vi "code-generator.vi"() -> ()   [LabVIEW 2014]
uses:
  <vilib>/addons/Digital Filter Design/_Objects.llb/DFD Quantization Settings.ctl
  <vilib>/addons/Digital Filter Design/_Objects.llb/DFD Quantization Sources.ctl
  <vilib>/addons/Digital Filter Design/FXPModel.llb/DFD FXP Quantize Coef (Easy).vi
  <vilib>/addons/Digital Filter Design/Process.llb/DFD Filtering (Wfm).vi
  <vilib>/addons/Digital Filter Design/FXPLib.llb/DFD FXP to I16 (scalar).vi
  <vilib>/addons/Digital Filter Design/CodeGen.llb/DFD FXP C Code Generator.vi
  <vilib>/Utility/VariantDataType/GetNumericFxpInfo.vi
  <vilib>/addons/Digital Filter Design/FXPSim.llb/dfd_Check Input FXP Settings.vi
  <vilib>/addons/Digital Filter Design/FXPSim.llb/dfd_Check SRate Simulation Integer Input.vi
  <vilib>/addons/Digital Filter Design/FXPSim.llb/dfd_FXP Simu.vi
  <vilib>/addons/Digital Filter Design/_Objects.llb/DFD FXP Statistics Data.ctl
  <vilib>/addons/Digital Filter Design/FXPSim.llb/SimXnode/DFD FXP Simulation.xnode
  <vilib>/addons/Digital Filter Design/_Objects.llb/DFD Filter Obj.ctl
  <vilib>/addons/Digital Filter Design/_Objects.llb/DFD Filter Coef.ctl
  <vilib>/addons/Digital Filter Design/_Objects.llb/DFD Filter Structure Type Selector.ctl
  <vilib>/addons/Digital Filter Design/_Objects.llb/dfd_Internal Quantization Settings.ctl
  <vilib>/addons/Digital Filter Design/_Objects.llb/dfd_Internal Quantization Srcs.ctl
  <vilib>/addons/Digital Filter Design/_Objects.llb/DFD Coef Norm Type.ctl
  <vilib>/addons/Digital Filter Design/NI_DigFilterLicensed.lvlib
  <vilib>/measure/NI_MABase.lvlib
  <vilib>/addons/Digital Filter Design/NI_DigFilter_FXP.lvlib
  <vilib>/Utility/VariantDataType/VariantType.lvlib
panel:
  out "output files":path[](array[path])
  out "coefficients report":string
  out "filtering text report":string
  out "signal out":waveform(dbl)[](graph)
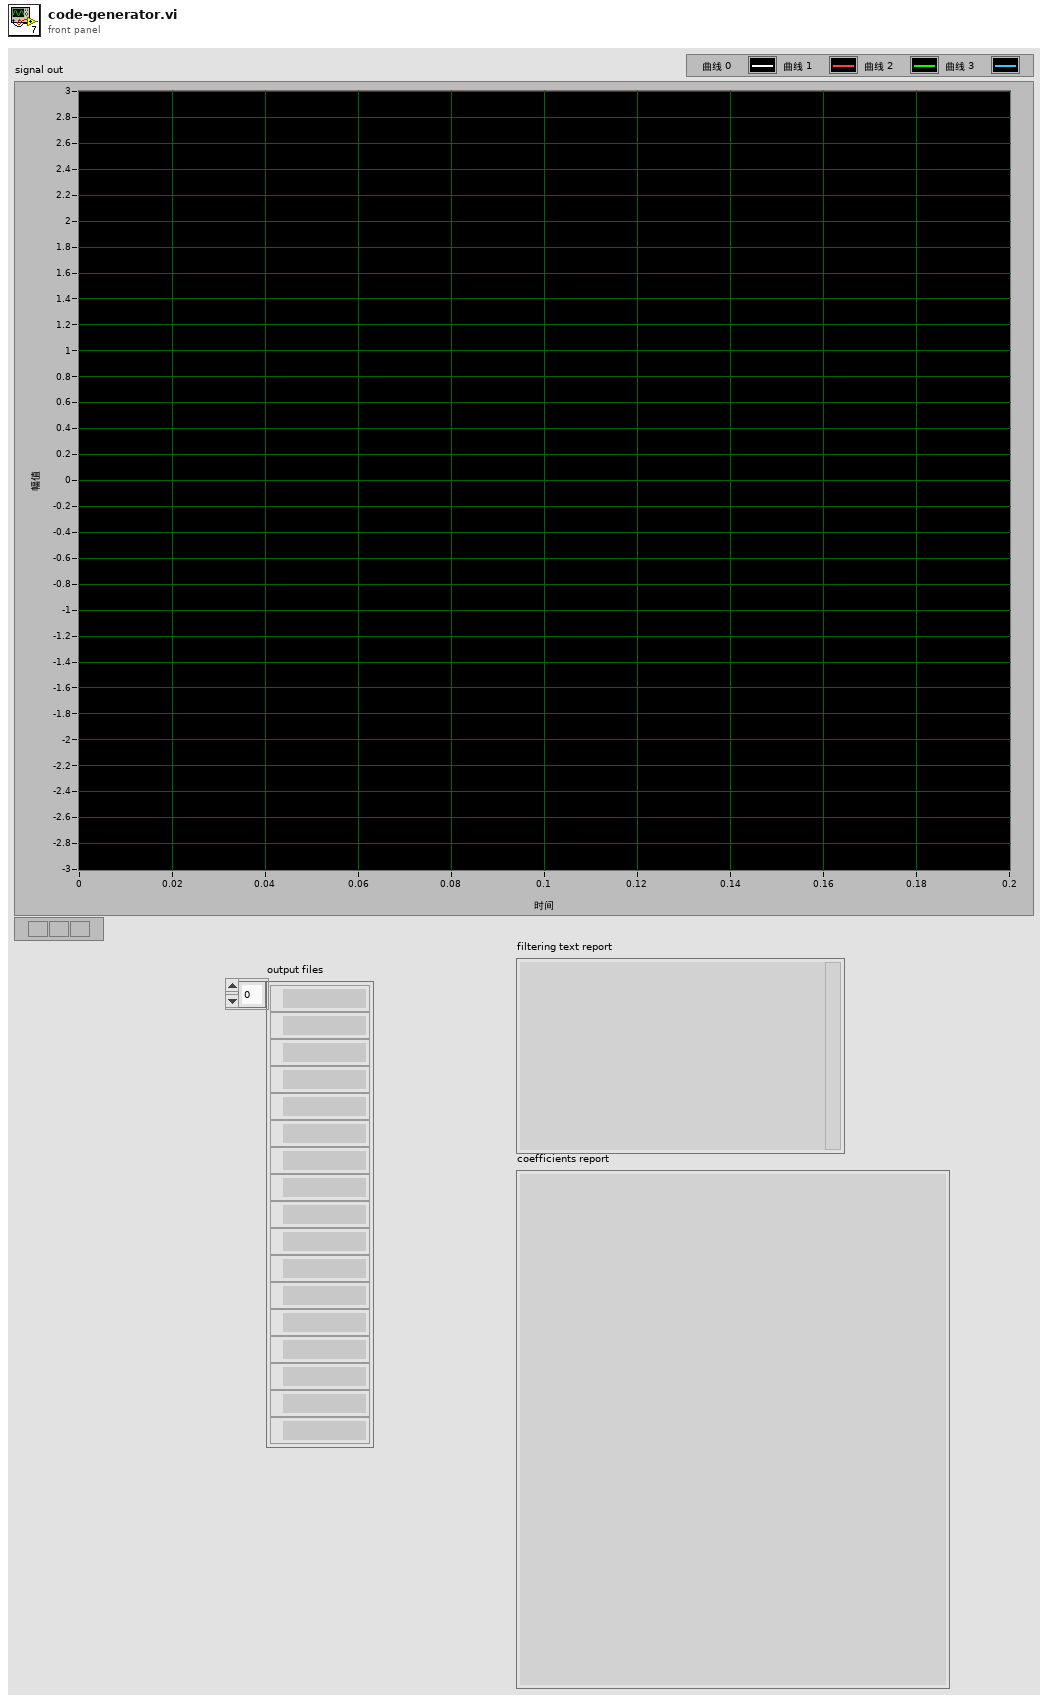
[diagram p1: front panel]
types:
  T1 = cluster{"gain processing":u16, "gain word length":i16}
  T2 = cluster{"frequency":dbl, "amplitude":dbl, "phase":dbl}[]
  T3 = enum16{"Lowpass", "Highpass", "Bandpass", "Bandstop"}
  T4 = typedef "NI_DigFilterLicensed.lvlib/DFD Quantization Settings.ctl" = cluster{"source":T5, "wl":i16, "iwl":i16, "overflow mode":enum16{"Saturation", "Wrap"}, "rounding mode":enum16{"Nearest", "Truncation"}, "signed?":bool}
  T5 = typedef "NI_DigFilterLicensed.lvlib/DFD Quantization Sources.ctl" = u16
  T6 = typedef "NI_DigFilterLicensed.lvlib/DFD Filter Obj.ctl" = cluster{"mSRate_Fs":dbl, "mSRate_Version":string, "mSRate_Comments":string, "mSRate_OrgCoef":T7, "mSRate_CurCoef":T7, "mSRate_Quantized?":bool, "mSRate_QCoef":T7, "mSRate_QSettings":T9[], "mSRate_Order":i32, "mSRate_Scaling":cluster{"mSRate_ScaleByPowerOf2?":bool, "mSRate_ScaleType":T11}}
  T7 = typedef "NI_DigFilterLicensed.lvlib/DFD Filter Coef.ctl" = cluster{"type":T8, "gain":dbl, "coef a (k)":dbl[], "coef b (v)":dbl[]}
  T8 = typedef "NI_DigFilterLicensed.lvlib/DFD Filter Structure Type Selector.ctl" = enum16{"Undefined", "FIR Direct Form", "FIR Direct Form Transposed", "FIR Symmetric", "FIR Antisymmetric", "IIR Direct Form I", "IIR Direct Form I Transposed", "IIR Direct Form II", "IIR Direct Form II Transposed", "IIR Cascaded Second Order Sections Form I", "IIR Cascaded Second Order Sections Form I Transposed", "IIR Cascaded Second Order Sections Form II", "IIR Cascaded Second Order Sections Form II Transposed", "Lattice Allpass (basic sections)", "Lattice Allpass (one multiplier sections)", "Lattice Allpass (normalized sections)", "Lattice AR (basic sections)", "Lattice AR (one multiplier sections)", "Lattice AR (normalized sections)", "Lattice MA (minimum phase)", "Lattice MA (maximum phase)", "Lattice ARMA (basic sections)", "Lattice ARMA (one multiplier sections)", "Lattice ARMA (normalized sections)"}
  T9 = typedef "NI_DigFilterLicensed.lvlib/dfd_Internal Quantization Settings.ctl" = cluster{"source":T10, "wl":i16, "iwl":i16, "overflow mode":enum16{"Saturation", "Wrap"}, "rounding mode":enum16{"Nearest", "Truncation"}, "signed?":bool}
  T10 = typedef "NI_DigFilterLicensed.lvlib/dfd_Internal Quantization Srcs.ctl" = u16
  T11 = typedef "NI_DigFilterLicensed.lvlib/DFD Coef Norm Type.ctl" = enum16{"No Norm", "Time Domain 1-Norm", "Time Domain 2-Norm", "Time Domain Inf-Norm"}
  T12 = typedef "NI_DigFilterLicensed.lvlib/DFD FXP Statistics Data.ctl" = cluster{"max value":ext, "min value":ext, "#overflows":i32, "#underflows":i32, "#operations":i32}
  T13 = cluster{"quantizer source":T5, "statistics information":T12}[]
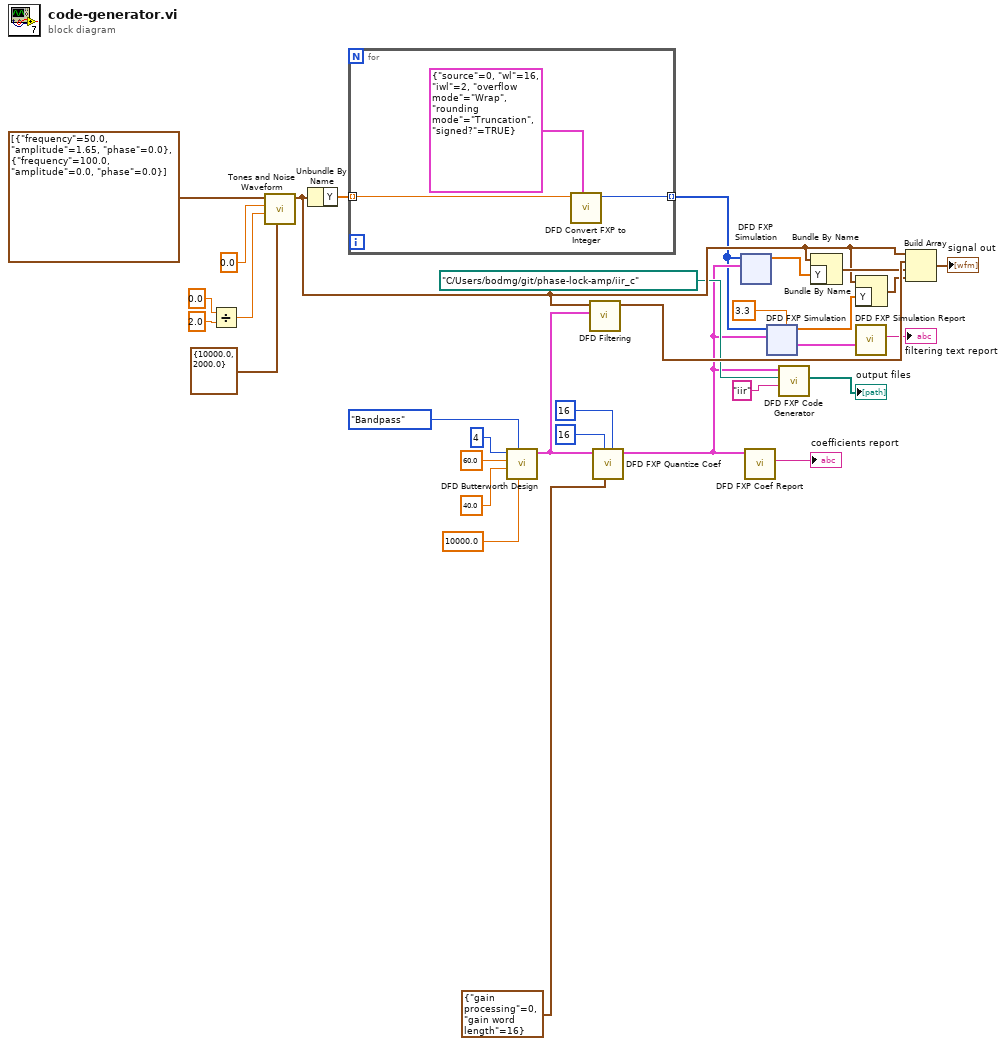
[diagram p0: block diagram]
diagram:
  n1 = Divide(x=0.0 ("offset"), y=2.0) -> (x/y=w17:dbl)
  n2 = call <vilib>:"Tones and Noise Waveform.vi"("sampling info"=cluster{"Fs":dbl, "#s":dbl} {"Fs"=10000.0, "#s"=2000.0}, "offset"=w17, "noise (rms)"=0.0, "tones"=T2 [{"frequency"=50.0, "amplitude"=1.65, "phase"=0.0}, {"frequency"=100.0, "amplitude"=0.0, "phase"=0.0}]) -> ("signal out"=w9:waveform(dbl))  [unwired: 6 in, 1 out]
  n3 = Unbundle By Name(w9) -> ("Y"=w2:dbl[])
  n4 = for {
    tunnel: w2 -> [w35] mode=indexing
    tunnel: [w34] -> w1 mode=indexing
    n5 = call-poly <vilib>:"DFD Convert FXP to Integer.vi"("quantization settings"=T4 {"source"=0, "wl"=16, "iwl"=2, "overflow mode"=enum."Wrap", "rounding mode"=enum."Truncation", "signed?"=TRUE}, "FXP value"=w35) -> ("I16"=w34:i16)  [unwired: 8 in, 1 out]
  }
  n6 = call <vilib>:"DFD Butterworth Design.vi"("fs [Hz]"=10000.0, "filter type"=T3."Bandpass", "low cutoff freq [Hz]"=40.0, "high cutoff freq [Hz]"=60.0, "order"=4) -> ("filter out"=w22:T6)  [unwired: 5 in, 1 out]
  n7 = call-poly <vilib>:"DFD Filtering.vi"("filter"=w22, "signal in"=w9) -> ("signal out"=w24:waveform(dbl))  [unwired: 8 in, 1 out]
  n8 = call-poly <vilib>:"DFD FXP Quantize Coef.vi"("coefficients b/v word length"=i16 16, "gain settings"=T1 {"gain processing"=0, "gain word length"=16}, "coefficients a/k word length"=i16 16, "filter in"=w22) -> ("filter out"=w3:T6)  [unwired: 6 in, 1 out]
  n9 = xnode "DFD FXP Simulation"("filter in"=w3, "signal in"=w1) -> ("DBL signal out"=w19:dbl[])  [unwired: 4 in, 3 out]
  n10 = call <vilib>:"DFD FXP Coef Report.vi"("filter in"=w3) -> ("coefficients report"=→"coefficients report":string)  [unwired: 8 in, 2 out]
  n11 = xnode "DFD FXP Simulation"("input range"=3.3, "filter in"=w3, "signal in"=w1) -> ("filtering statistics report"=w12:T13, "DBL signal out"=w14:dbl[])  [unwired: 3 in, 2 out]
  n12 = call-poly <vilib>:"DFD FXP Code Generator.vi"("filter name"="iir", "destination folder"=path "C:/Users/bodmg/git/phase-lock-amp/iir_c", "filter in"=w3) -> ("output files"=→"output files":path[])  [unwired: 7 in, 1 out]
  n13 = Bundle By Name(cluster=w9, "Y"=w19) -> (w13:waveform(dbl))
  n14 = Bundle By Name(cluster=w9, "Y"=w14) -> (w8:waveform(dbl))
  n15 = call <vilib>:"DFD FXP Simulation Report.vi"("filtering statistics report"=w12) -> ("filtering text report"=→"filtering text report":string)  [unwired: 9 in, 1 out]
  n16 = Build Array(w9, w24, w13, w8) -> (→"signal out":waveform(dbl)[])
